vi "test_suite_run.vi"() -> ()   [LabVIEW 2009]
uses:
  protocol_Generic/Protocol_Generic.lvclass
  protocol_A/Protocol_a.lvclass
  protocol_B/Protocol_B.lvclass
panel:
  out "error out":errorcluster
  in  "error in (no error)":errorcluster
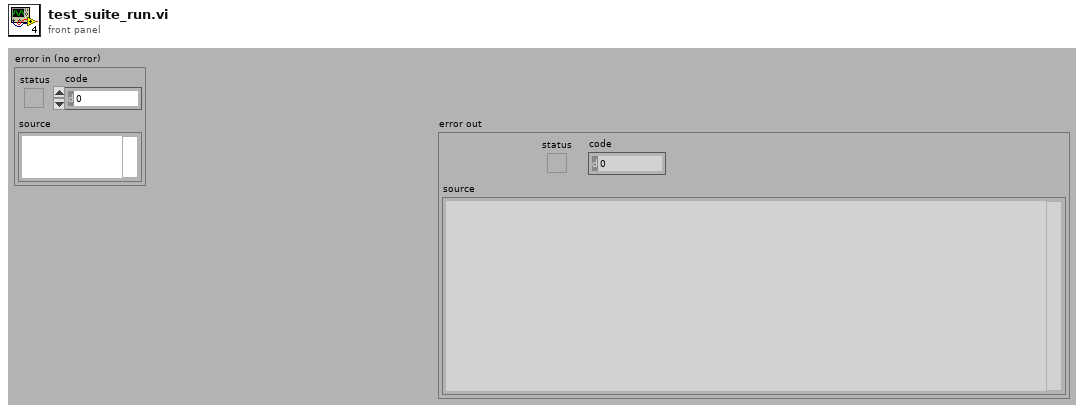
[diagram p1: front panel]
types:
  T1 = cluster{"Protocol_Generic.lvclass":refnum<class "Protocol_Generic.lvclass">}[]
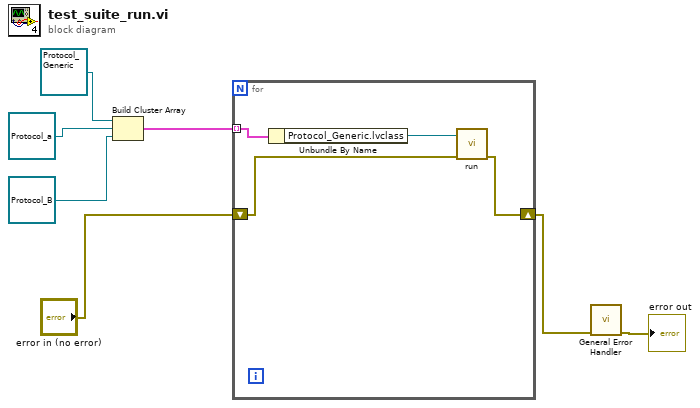
[diagram p0: block diagram]
diagram:
  n1 = Build Cluster Array(refnum<class "Protocol_Generic.lvclass"> refnum ("Protocol_Generic.lvclass"), refnum<class "Protocol_a.lvclass"> refnum ("Protocol_A.lvclass"), refnum<class "Protocol_B.lvclass"> refnum ("Protocol_B.lvclass")) -> (w3:T1)
  n2 = for {
    tunnel: w3 -> [w11] mode=indexing
    shift-right: [w8] -> w1
    shift-left: "error in (no error)" -> [w9]
    n3 = Unbundle By Name(w11) -> ("Protocol_Generic.lvclass"=w10:refnum<class "Protocol_Generic.lvclass">)
    n4 = call-dynamic "run.vi"("error in (no error)"=w9, "Protocol_Generic in"=w10) -> ("error out"=w8:errorcluster)  [unwired: 8 in, 1 out]
  }
  n5 = call <vilib>:"General Error Handler.vi"("error in (no error)"=w1) -> ("error out"=→"error out":errorcluster)  [unwired: 10 in, 4 out]
